vi "UI Page Disply_Error Occur.vi"(8 "error in (no error)":errorcluster, 10 "Tab Main":refnum<vi>, 11 "Main Class in":refnum<class "Main Class.lvclass">) -> (0 "error out":errorcluster, 3 "Main Class out":refnum<class "Main Class.lvclass">)   [LabVIEW 2019, in "Main Class.lvclass"]
uses:
  Main Class.lvclass
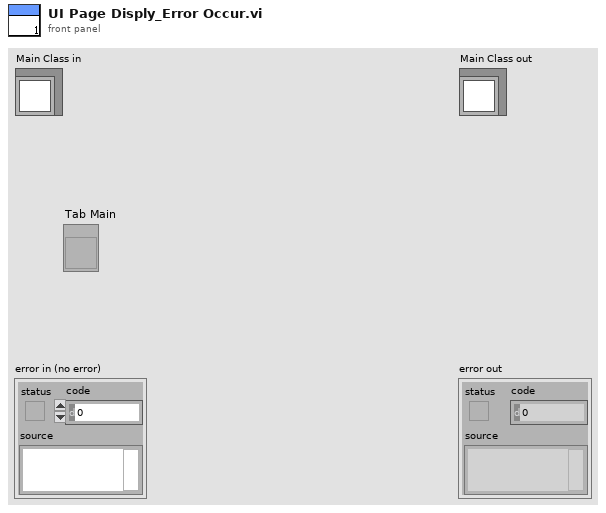
[diagram p1: front panel]
types:
  T1 = enum32{"Main", "Project", "Set", "IO", "Step", "ErrMsg", "MsgLog", "ProductCollect", "AdStatus"}
  T2 = enum32{"Main", "Project", "Set", "IO", "Robot", "ErrMsg", "MsgLog", "ProductCollect", "AdStatus"}
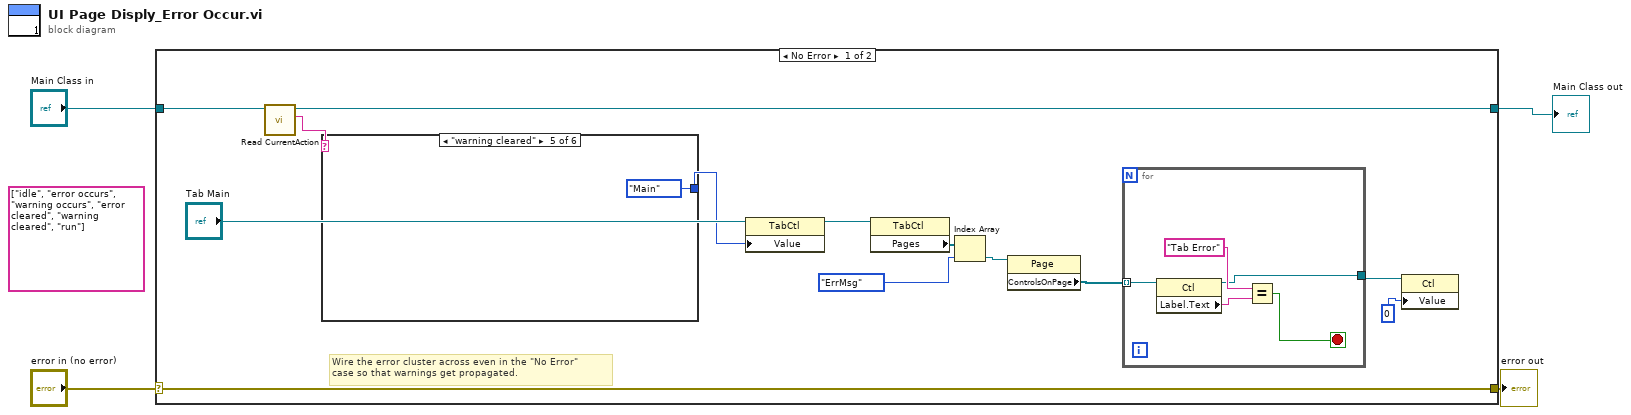
[diagram p0: block diagram]
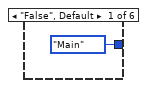
[diagram p2: hidden frame]
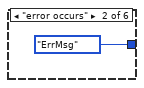
[diagram p3: hidden frame]
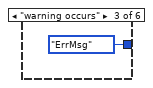
[diagram p4: hidden frame]
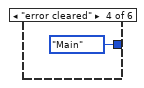
[diagram p5: hidden frame]
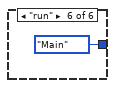
[diagram p6: hidden frame]
diagram:
  (unwired) string[] ["idle", "error occurs", "warning occurs", "error cleared", "warning cleared", "run"] ("Array")
  n1 = case shown="No Error" "error in (no error)" {
    selector: "error in (no error)" -> [w17 w30]
    tunnel: [w17 w30] -> w3
    tunnel: [w15 w29] -> w1
    tunnel: "Main Class in" -> [w16 w29]
    frame No Error {
      # "Wire the error cluster across even in the \"No Error\"\ncase so that warnings get propagated."
      n2 = call-dynamic "Read CurrentAction.vi"("Main Process Class in"=w16) -> ("CurrentAction"=w14:string, "Main Process Class out"=w15:refnum<class "Main Class.lvclass">)  [unwired: 8 in, 1 out]
      n3 = case shown="\"warning cleared\"" w14 {
        tunnel: [T2."Main" ("Tab Main") T2."ErrMsg" ("Tab Main") T2."ErrMsg" ("Tab Main") T2."Main" ("Tab Main") T1."Main" ("Tab Main") T2."Main" ("Tab Main")] -> w12
        frame "False", Default {
        }
        frame "error occurs" {
        }
        frame "warning occurs" {
        }
        frame "error cleared" {
        }
        frame "warning cleared" {
        }
        frame "run" {
        }
      }
      n4 = property class="TabCtl"(reference="Tab Main", "Value"=w12) -> (reference out=w11:refnum<vi>)  [unwired: 1 in, 1 out]
      n5 = property class="TabCtl"(reference=w11) -> ("Pages"=w10:refnum<vi>[])  [unwired: 1 in, 2 out]
      n6 = Index Array(array=w10, index=T1."ErrMsg" ("Tab Main")) -> (element=w8:refnum<vi>)
      n7 = property class="Page"(reference=w8) -> ("ControlsOnPage"=w7:refnum<vi>[])  [unwired: 1 in, 2 out]
      n8 = for {
        tunnel: w7 -> [w22] mode=indexing
        tunnel: [w18] -> w6
        stop <- w19 stop-if-true
        n9 = property class="Ctl"(reference=w22) -> (reference out=w18:refnum<vi>, "Label.Text"=w21:string)  [unwired: 1 in, 1 out]
        n10 = Equal?(x="Tab Error", y=w21) -> (x = y?=w19:bool)
      }
      n11 = property class="Ctl"(reference=w6, "Value"=0) -> ()  [unwired: 1 in, 2 out]
    }
    frame Error {
    }
  }
  "error out" <- w3
  "Main Class out" <- w1
